vi "AlliGator Extrapolate Decay.vi"(8 "error in (no error)":errorcluster, 9 "Replace Plot (T)?":bool=TRUE, 11 "Selected Plot Info":T1={"Multiplot XY Graph"=refnum, "Mouse Coordinates"={"Horizontal"=0, "Vertical"=0}, "Plot Index"=-1}) -> (0 "Error Out":errorcluster, 1 "Message":string, 3 "Extrapolated Decay":cluster{"t Array":dbl[], "IRF Array":dbl[]})   [LabVIEW 2021, in "AlliGator Decay Preprocessing.lvlib"]
doc: "Extrapolates a truncated decay by trying to fit an exponential to the tail part and connect it to the head part ."
uses:
  AlliGator Decay Preprocessing.lvlib
  Graphs/XY Graph/XY Graph Selected Plot Info.ctl
  Graphs/XY Graph/XY Graph Refnum.ctl
  <vilib>/Utility/miscctls.llb/LVPoint32TypeDef.ctl
  Settings/AlliGator Settings List.ctl
  Variant/Variant to Data/Variant to DBL.vi
  Variant/Variant to Data/Variant to U32.vi
  Variant/Variant to Data/Variant to Boolean.vi
  Settings/AlliGator Settings.lvlib
  Graphs/XY Graph/XY Graph Add-Ons.lvlib
  Variant/Variant to Data/Variant to Data.lvlib
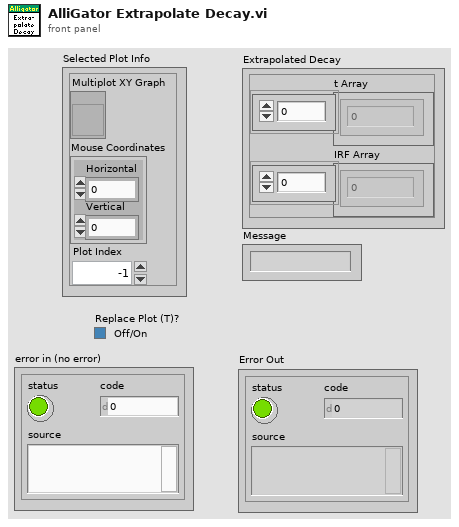
[diagram p1: front panel]
types:
  T1 = typedef "XY Graph Add-Ons.lvlib/XY Graph Selected Plot Info.ctl" = cluster{"Multiplot XY Graph":T2, "Mouse Coordinates":T3, "Plot Index":i32}
  T2 = typedef "XY Graph Add-Ons.lvlib/XY Graph Refnum.ctl" = refnum<vi>
  T3 = typedef "LVPoint32TypeDef.ctl" = cluster{"Horizontal":i32, "Vertical":i32}
  T4 = typedef "AlliGator Settings.lvlib/AlliGator Settings List.ctl" = enum16{"GUI:Visible Settings Tab", "GUI:Last Run Version", "Source Image:Use Image Histogram for Contrast", "Source Image:Low Count Pixels Rejection Options", "Source Image:High Count Pixels Rejection Options", "Source Image:Use Image Brightness", "Source Image:Blend Overlay with Image Background", "Source Image:Use Fixed ROI Diameter", "Source Image:ROI Diameter", "Source Image:ROI Center Color", "Source Image:Peak Threshold", "Source Image:Intensity Threshold", "Source Image:Image Binning Options", "Source Image:Image Smoothing Options", "Source Image:Image Histogram Active", "Source Image:Invert Binary Mask", "Source Image:Hot Pixel Removal", "Source Image:Overlay Analyzed ROI Center", "Source Image:Auto-Adjust Contrast", "Source Image:Histogram Lower Percentile", "Source Image:Histogram Upper Percentile", "Source Image:Save Source Image", "Source Image:Scale Bar Options", "Source Image:Image Resolution (Pixel Size)", "Source Image:Flatfield Correction", "Source Image:Show Dead Left Columns Correction", "Source Image:Dead Left Columns Correction", "Source Image:Image Pre-Processing Operations Order", "Source Image:Overlay ROI Median", "Source Image:Median Overlay Color", "Data Information:Gate Width", "Data Information:Nanotime Gate Separation", "Data Information:Macrotime Gate Separation", "Data Information:Gate Step", "Data Information:# Gates", "Data Information:Gate Image Exposure", "Data Information:Gate Image Integration", "Data Information:Gates to Skip", "Data Information:Gates to Keep", "Data Information:Define Gates to", "Data Information:Channel Name", "Data Information:Available Channel Names", "Data Information:Channel Arithmetic", "Data Information:Background File Subtraction", "Data Information:Background File", "Data Information:Background Scaling Factor", "Data Information:Background Pile-up Correction", "Data Information:Background Pixel Well Capacity", "Data Information:Laser Period", "Data Information:SYNC Period", "Data Information:Pile-up Correction", "Data Information:Pixel Well Capacity", "Data Information:Dataset Scaling Factor", "Fluorescence Decay_Decay Pre-Processing:Reverse Gates", "Fluorescence Decay_Decay Pre-Processing:Verbose Decay Pre-Processing", "Fluorescence Decay_Decay Pre-Processing:Use Decay Pre-Processing", "Fluorescence Decay_Decay Pre-Processing:Background Subtraction", "Fluorescence Decay_Decay Pre-Processing:Background Definition Range", "Fluorescence Decay_Decay Pre-Processing:Baseline Subtraction Method", "Fluorescence Decay_Decay Pre-Processing:Decay Pre-Processing Operations Order", "Fluorescence Decay_Decay Pre-Processing:Smoothing Parameter", "Fluorescence Decay_Decay Pre-Processing:Shift Decay", "Fluorescence Decay_Decay Pre-Processing:Decay Shift Parameters", "Fluorescence Decay_Decay Pre-Processing:Fold Decay", "Fluorescence Decay_Decay Pre-Processing:# Folds", "Fluorescence Decay_Decay Pre-Processing:1-Normalize Decay", "Fluorescence Decay_Decay Pre-Processing:[0-1]-Normalize Decay", "Fluorescence Decay_Decay Pre-Processing:Smoothen Decay", "Fluorescence Decay_Decay Pre-Processing:Extrapolate Decay", "Fluorescence Decay_Decay Pre-Processing:Use Periodicity", "Fluorescence Decay_Decay Pre-Processing:Use Cursors", "Fluorescence Decay_Decay Pre-Processing:Tail Fraction", "Fluorescence Decay_Decay Pre-Processing:Head Fraction", "Fluorescence Decay_Decay Pre-Processing:Additional Points", "Fluorescence Decay_Decay Pre-Processing:Straighten Decay", "Fluorescence Decay_Decay Pre-Processing:Constant Background", "Fluorescence Decay_Decay Pre-Processing:Pixel-Normalize Decay", "Fluorescence Decay_Advanced Analysis:Extract IRF instead of Decay", "Fluorescence Decay_Advanced Analysis:IRF Extraction Options", "Fluorescence Decay_Advanced Analysis:IRF Optimization Options", "Fluorescence Decay_Advanced Analysis:Square Pulse Options", "Fluorescence Decay_Advanced Analysis:IRF Order", "Fluorescence Decay_Advanced Analysis:IRF Time Constants", "Fluorescence Decay_Advanced Analysis:Wavelet Analysis Options", "Fluorescence Decay_Advanced Analysis:Average Lifetime Options", "Fluorescence Decay_Fit Options:Fit Options", "Fluorescence Decay_Fit Options:Use Legacy Fitting Approach", "Fluorescence Decay_Fit Options:Use Data Information Laser Period", "Fluorescence Decay_Fit Parameters:Displayed Fit Parameters", "Fluorescence Decay_Fit Parameters:Fit Parameter Constraints", "Fluorescence Decay_Fit Parameters:Export Tabulated Results", "Fluorescence Decay_Fit Parameters:MLE Baseline Offset Type", "Fluorescence Decay_Fit Parameters:MLE Baseline Offset", "Fluorescence Decay_Fit Parameters:Guess Parameter Names", "Fluorescence Decay_Fit Parameters:Guess Parameter Values", "Fluorescence Decay_Fit Parameters:Guess Parameters Options", "Fluorescence Decay_Styles:Show Last Decay Only", "Fluorescence Decay_Styles:Decay Graph Color Array", "Fluorescence Decay:Decay Graph Active", "Fluorescence Decay Statistics:Min Peak Value", "Fluorescence Decay Statistics:Reject Low Decay Peak Pixels", "Fluorescence Decay Statistics:Reject High Decay Peak Pixels", "Fluorescence Decay Statistics:Max Peak Value", "Time Traces:Use File Timestamp", "Time Traces:Time Step", "Time Traces:Use Intensity Correction File", "Time Traces:Intensity Correction File", "Phasor Plot:Phasor Plot Smoothing Options", "Phasor Plot:Phasor Plot Size", "Phasor Plot:Phasor Plot Graphics Options", "Phasor Plot:Cumulative Phasor Plot", "Phasor Plot:Use Phasor Brightness", "Phasor Plot:Blend Overlay with Phasor Background", "Phasor Plot:Save Phasor Plot", "Phasor Plot:Show References", "Phasor Plot:Phasor Ratio Decay Range", "Phasor Plot:Exponential Fading", "Phasor Plot:Phasor Ratio Reference Colors", "Phasor Plot:Reference Radius", "Phasor Plot:Show Color Map Vertices", "Phasor Plot:Phasor Plot Active", "Phasor Plot:Phasor Ratio Color Map Type", "Phasor Plot:Phasor Ratio Color Map", "Phasor Plot:Phasor Ratio Display Range", "Phasor Plot:Selected Image ROI(s)", "Phasor Plot:All Image ROIs", "Phasor Plot:Selected Phasor Plot ROI(s)", "Phasor Plot:All Phasor Plot ROIs", "Phasor Plot:Phasor Ratio Color-Coded Quantity", "Phasor Plot:Store Phasor Harmonics", "Phasor Plot:Draw Reference Segment", "Phasor Plot:User-Defined Quantity", "Phasor Graph:Phasor Frequency", "Phasor Graph:Phasor Ratio Type", "Phasor Graph:Pixel-level Phasor Computation", "Phasor Graph:Save Phasor Graph", "Phasor Graph:Phasor Graph Active", "Phasor Graph:Phasor SDV Options", "Phasor Calibration:Use Backup Calibration if needed", "Phasor Graph:Define Shortest Lifetime as", "Phasor Calibration:Backup Calibration Type", "Phasor Calibration:Calibration Type", "Phasor Calibration:Calibration Lifetime", "Phasor Calibration:Calibration Map Algorithm", "Single-Exponential Phasor Locus (SEPL):Gate Parameters", "Single-Exponential Phasor Locus (SEPL):User-defined Gate", "Single-Exponential Phasor Locus (SEPL):User-defined IRF", "Single-Exponential Phasor Locus (SEPL):Phasor Parameters", "Single-Exponential Phasor Locus (SEPL):Decay & IRF Parameters", "Single-Exponential Phasor Locus (SEPL):Display Parameters", "Lifetime Analysis:Decay Analysis Parameters", "Lifetime Analysis:Lifetime Map Active", "Plugins:Python Settings", "Miscellaneous:Verbose Mode", "Miscellaneous:Beep after Script", "Miscellaneous:Saved Image File Format", "Miscellaneous:Exported Gate Image Settings", "Miscellaneous:Include Loading in Timing", "Miscellaneous:Verbose Settings Mode", "Miscellaneous:Histogram Options", "Miscellaneous:Beep on Error", "Miscellaneous:# Logical Processors Used", "Miscellaneous:ROI Description Max Characters", "Miscellaneous:Verbose Error Mode", "Miscellaneous:Transparent Mask Color"}
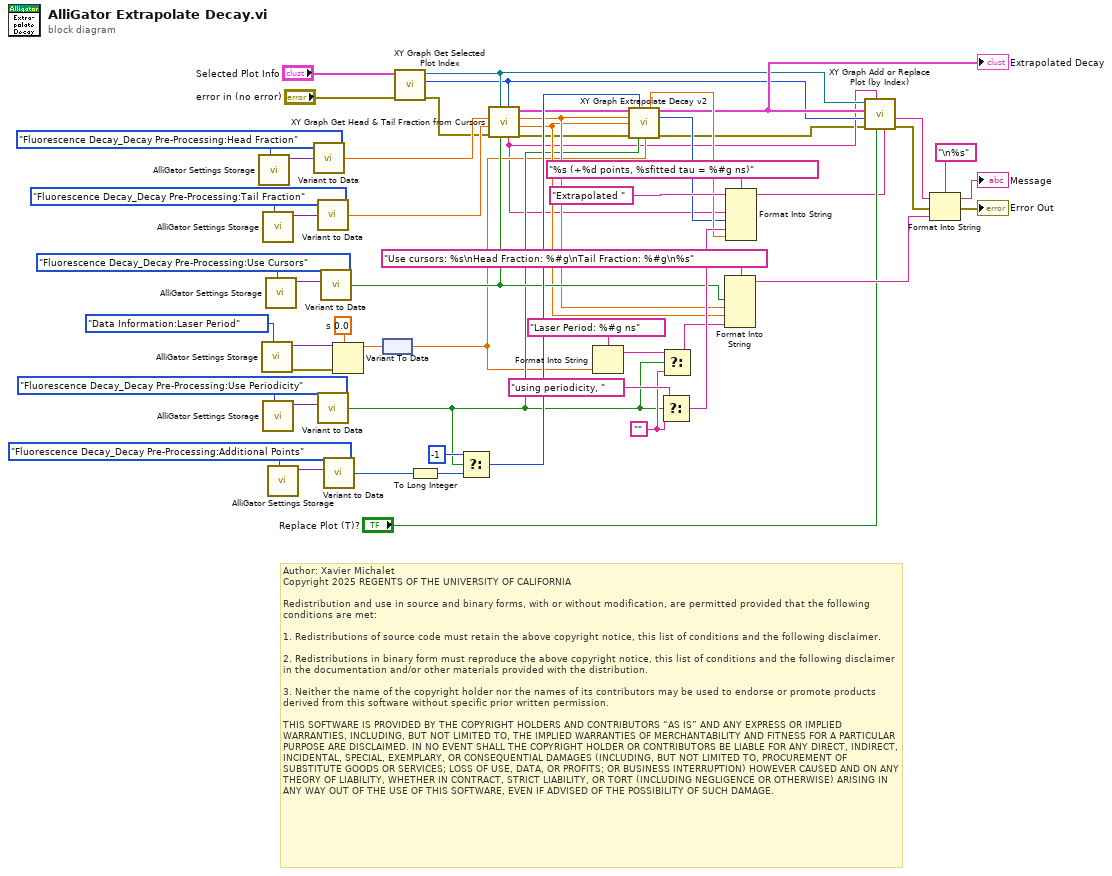
[diagram p0: block diagram]
diagram:
  w41 = dbl[unit] 0.0  # s
  w22 = ""
  # "Author: Xavier Michalet\nCopyright 2025 REGENTS OF THE UNIVERSITY OF CALIFORNIA\n\nRedistribution and use in source and binary forms, with or without modification, are permitted provided that the following conditions are met:\n\n1. Redistributions of source code must retain the above copyright notice, this list of conditions and the following disclaimer.\n\n2. Redistributions in binary form must reproduce the above copyright notice, this list of conditions and the following disclaimer in the documentation and/or other materials provided with the distribution.\n\n3. Neither the name of the copyright holder nor the names of its contributors may be used to endorse or promote products derived from this software without specific prior written permission.\n\nTHIS SOFTWARE IS PROVIDED BY THE COPYRIGHT HOLDERS AND CONTRIBUTORS “AS IS” AND ANY EXPRESS OR IMPLIED WARRANTIES, INCLUDING, BUT NOT LIMITED TO, THE IMPLIED WARRANTIES OF MERCHANTABILITY AND FITNESS FOR A PARTICULAR PURPOSE ARE DISCLAIMED. IN NO EVENT SHALL THE COPYRIGHT HOLDER OR CONTRIBUTORS BE LIABLE FOR ANY DIRECT, INDIRECT, INCIDENTAL, SPECIAL, EXEMPLARY, OR CONSEQUENTIAL DAMAGES (INCLUDING, BUT NOT LIMITED TO, PROCUREMENT OF SUBSTITUTE GOODS OR SERVICES; LOSS OF USE, DATA, OR PROFITS; OR BUSINESS INTERRUPTION) HOWEVER CAUSED AND ON ANY THEORY OF LIABILITY, WHETHER IN CONTRACT, STRICT LIABILITY, OR TORT (INCLUDING NEGLIGENCE OR OTHERWISE) ARISING IN ANY WAY OUT OF THE USE OF THIS SOFTWARE, EVEN IF ADVISED OF THE POSSIBILITY OF SUCH DAMAGE."
  n1 = call "AlliGator Settings Storage.vi"("AlliGator Settings List"=AlliGator_Settings_List."Fluorescence Decay_Decay Pre-Processing:Head Fraction") -> ("Variant Data out"=w30:variant)  [unwired: 9 in, 1 out]
  n2 = call "AlliGator Settings Storage.vi"("AlliGator Settings List"=AlliGator_Settings_List."Data Information:Laser Period") -> ("Error Out"=w42:errorcluster, "Variant Data out"=w43:variant)  [unwired: 9 in]
  n3 = call "AlliGator Settings Storage.vi"("AlliGator Settings List"=AlliGator_Settings_List."Fluorescence Decay_Decay Pre-Processing:Tail Fraction") -> ("Variant Data out"=w50:variant)  [unwired: 9 in, 1 out]
  n4 = call "AlliGator Settings Storage.vi"("AlliGator Settings List"=AlliGator_Settings_List."Fluorescence Decay_Decay Pre-Processing:Use Periodicity") -> ("Variant Data out"=w48:variant)  [unwired: 9 in, 1 out]
  n5 = call "AlliGator Settings Storage.vi"("AlliGator Settings List"=AlliGator_Settings_List."Fluorescence Decay_Decay Pre-Processing:Use Cursors") -> ("Variant Data out"=w34:variant)  [unwired: 9 in, 1 out]
  n6 = call "AlliGator Settings Storage.vi"("AlliGator Settings List"=AlliGator_Settings_List."Fluorescence Decay_Decay Pre-Processing:Additional Points") -> ("Variant Data out"=w49:variant)  [unwired: 9 in, 1 out]
  n7 = call-poly "Variant to Data.vi"("Variant"=w30) -> ("Value"=w28:dbl)  [unwired: 8 in]
  n8 = call-poly "Variant to Data.vi"("Variant"=w50) -> ("Value"=w31:dbl)  [unwired: 8 in]
  n9 = call-poly "Variant to Data.vi"("Variant"=w48) -> ("Value"=w20:bool)  [unwired: 8 in]
  n10 = call-poly "Variant to Data.vi"("Variant"=w34) -> ("Value"=w26:bool)  [unwired: 8 in]
  n11 = call-poly "Variant to Data.vi"("Variant"=w49) -> ("Value"=w39:u32)  [unwired: 8 in]
  n12 = Variant To Data(error in=w42, type=w41, Variant=w43) -> (data=w40:dbl[unit])  [unwired: 1 out]
  n13 = node(w40) -> (w17:dbl)
  n14 = call "XY Graph Get Selected Plot Index.vi"("error in (no error)"="error in (no error)", "Selected Plot Info"="Selected Plot Info") -> ("error out"=w11:errorcluster, "Plot at Coordinates"=w8:i32, "XYGraph out"=w9:T2)  [unwired: 6 in, 1 out]
  n15 = To Long Integer(number=w39) -> (32bit integer=w27:i32)
  n16 = Select(t=-1, s=w20, f=w27) -> (s? t:f=w35:i32)
  n17 = call "XY Graph Get Head & Tail Fraction from Cursors.vi"("Active Plot Index"=w8, "Use Cursors"=w26, "XYGraph in"=w9, "error in (no error)"=w11, "Tail Fraction"=w31, "Head Fraction"=w28) -> ("error out"=w1:errorcluster, "Tail Fraction"=w23:dbl, "Head Fraction"=w24:dbl, "Plot out"=w32:cluster{"X Array":dbl[], "Y Array":dbl[]}, "Plot Name"=w3:string)  [unwired: 1 in]
  n18 = Format Into String(format string="Laser Period: %#g ns", w17) -> (resulting string=w18:string)  [unwired: 2 in, 1 out]
  n19 = call "XY Graph Extrapolate Decay v2.vi"("Plot in"=w32, "# Additional Points (-1: to Period)"=w35, "Head Fraction"=w24, "Tail Fraction"=w23, "Error In"=w1, "Periodic Decay"=w20, "Period"=w17) -> ("Fitted Tau"=w37:dbl, "Plot out"=w10:cluster{"X Array":dbl[], "Y Array":dbl[]}, "# Additional Points"=w36:i32, "error out"=w2:errorcluster)  [unwired: 3 in, 2 out]
  "Extrapolated Decay" <- w10
  n20 = Select(t="using periodicity, " ("initial string"), s=w20, f=w22) -> (s? t:f=w45:string)
  n21 = Select(t=w18, s=w20, f=w22) -> (s? t:f=w21:string)
  n22 = Format Into String(format string="Use cursors: %s\nHead Fraction: %#g\nTail Fraction: %#g\n%s", w26, w24, w23, w21) -> (resulting string=w14:string)  [unwired: 2 in, 1 out]
  n23 = Format Into String(format string="%s (+%d points, %sfitted tau = %#g ns)", initial string="Extrapolated ", w3, w36, w45, w37) -> (resulting string=w4:string)  [unwired: 1 in, 1 out]
  n24 = call "XY Graph Add or Replace Plot (by Index).vi"("New Plot Name"=w4, "Replace Plot (T)?"="Replace Plot (T)?", "Original Plot Name"=w3, "error in (no error)"=w2, "Plot Index"=w8, "Plot in"=w10, "XYGraph in"=w9) -> ("error out"=w7:errorcluster, "Message"=w6:string)  [unwired: 3 in]
  n25 = Format Into String(format string="\n%s", initial string=w6, error in=w7, w14) -> (resulting string=→"Message":string, error out=→"Error Out":errorcluster)
